vi "Write CorrOffset File.vi"(8 "error in":errorcluster, 10 "Offset Data In":T1(array[cluster]), 11 "File Path In":path) -> (0 "error out":errorcluster, 2 "Offset Data Out":T1(array[cluster]), 3 "File Path Out":path)   [LabVIEW 2020, in "GUCalibration2.lvlib"]
uses:
  GUCalibration2.lvlib
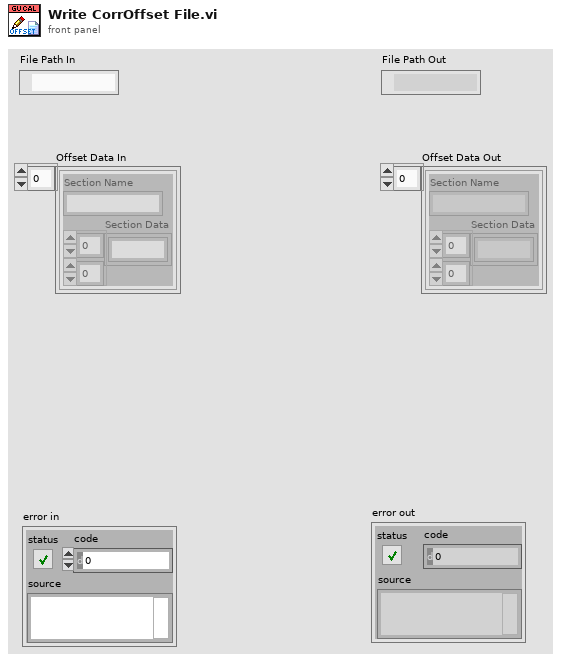
[diagram p1: front panel]
types:
  T1 = cluster{"Section Name":string, "Section Data":string[][]}[]
  T2 = enum16{"open", "replace", "create", "open or create", "replace or create", "replace or create with confirmation"}
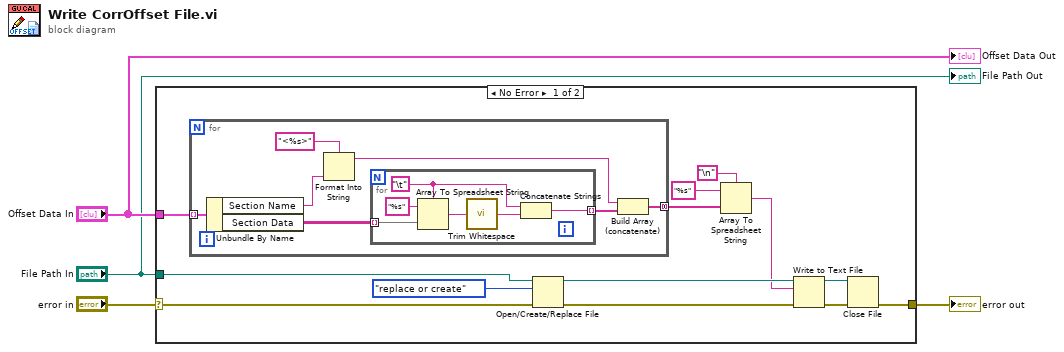
[diagram p0: block diagram]
diagram:
  n1 = case shown="No Error" "error in" {
    selector: "error in" -> [w7 w31]
    tunnel: [w8 w31] -> w4
    tunnel: "Offset Data In" -> [w6 _]
    tunnel: "File Path In" -> [w5 _]
    frame No Error {
      n2 = for {
        tunnel: w6 -> [w24] mode=indexing
        tunnel: [w20] -> w17 mode=concatenating
        n3 = Unbundle By Name(w24) -> ("Section Name"=w18:string, "Section Data"=w22:string[][])
        n4 = Format Into String(format string="<%s>", w18) -> (resulting string=w19:string)  [unwired: 2 in, 1 out]
        n5 = for {
          tunnel: w22 -> [w30] mode=indexing
          tunnel: [w25] -> w21 mode=indexing
          w26 = "\t"
          n6 = Array To Spreadsheet String(delimiter (Tab)=w26, array=w30, 3:"%s" ("format string")) -> (spreadsheet string=w28:string)
          n7 = call <vilib>:"Trim Whitespace.vi"("string"=w28) -> ("trimmed string"=w27:string)  [unwired: 1 in]
          n8 = Concatenate Strings(w26, w27) -> (w25:string)
        }
        n9 = Build Array (concatenate)(w19, w21) -> (w20:string[])
      }
      n10 = Open/Create/Replace File(file path (use dialog)=w5, error in=w7, operation (0:open)=T2."replace or create") -> (refnum out=w12:refnum<file>, error out=w13:errorcluster)  [unwired: 3 in, 1 out]
      n11 = Array To Spreadsheet String(delimiter (Tab)="\n", array=w17, 3:"%s" ("format string")) -> (spreadsheet string=w9:string)
      n12 = Write to Text File(file (use dialog)=w12, text=w9, error in=w13) -> (refnum out=w11:refnum<file>, error out=w10:errorcluster)  [unwired: 1 in, 1 out]
      n13 = Close File(refnum=w11, error in=w10) -> (error out=w8:errorcluster)  [unwired: 1 out]
    }
    frame Error {
    }
  }
  "error out" <- w4
  "File Path Out" <- "File Path In"
  "Offset Data Out" <- "Offset Data In"
